vi "camera get one frame-subvi.vi"(2 "error in":errorcluster, 3 "New Image":T2, 4 "Image Size":T1 {"V Bin" min=0.0; "H Bin" min=0.0 step=1.0}) -> (0 "error out":errorcluster, 1 "Image Out":T2)   [LabVIEW 2014]
uses:
  <vilib>/vision/Image Controls.llb/IMAQ Image.ctl
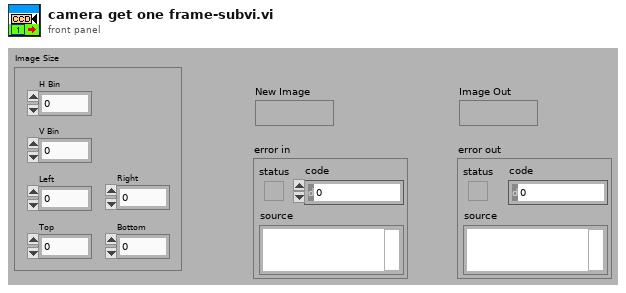
[diagram p1: front panel]
types:
  T1 = cluster{"H Bin":dbl, "V Bin":dbl, "Left":dbl, "Right":dbl, "Top":dbl, "Bottom":dbl}
  T2 = typedef "IMAQ Image.ctl" = refnum<image>
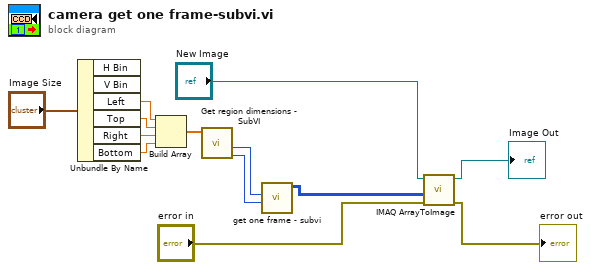
[diagram p0: block diagram]
diagram:
  n1 = Unbundle By Name("Image Size") -> ("Left"=w12:dbl, "Top"=w11:dbl, "Right"=w10:dbl, "Bottom"=w9:dbl)  [unwired: 2 out]
  n2 = Build Array(w12, w11, w10, w9) -> (w13:dbl[])
  n3 = call "Get region dimensions - SubVI.vi"("x1y1x2y2"=w13) -> ("y size"=w7:u64, "x size"=w8:u64)  [unwired: 7 in, 2 out]
  n4 = call "get one frame - subvi.vi"("Image Height"=w7, "Image Width"=w8) -> ("Image Array"=w3:i32[][])  [unwired: 9 in]
  n5 = call "IMAQ ArrayToImage"("error in (no error)"="error in", "Image Pixels (I16)"=w3, "Image"="New Image") -> ("error out"=→"error out":errorcluster, "Image Out"=→"Image Out":T2)  [unwired: 7 in]
